vi "rm.server.open visualizer.vi"(8 "error in (no error)":errorcluster, 11 "Device Ref in":T1 format="%.0x") -> (0 "error out":errorcluster, 3 "reference out":refnum<vi>)   [LabVIEW 2016, in "RM.Server.lvlib"]
uses:
  RM.Server.lvlib
  <vilib>/NI Veristand/Custom Device API/Custom Device Item Ref.ctl
  rm.server.visualize.vi
  <vilib>/NI VeriStand/Custom Device API/Custom Device API.lvlib
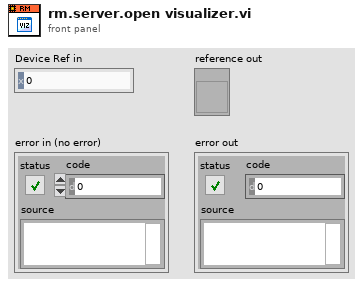
[diagram p1: front panel]
types:
  T1 = typedef "Custom Device API.lvlib/Custom Device Item Ref.ctl" = u64
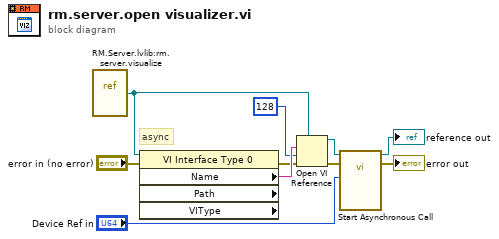
[diagram p0: block diagram]
diagram:
  # "async"
  n1 = vi-ref "RM.Server.lvlib:rm.server.visualize.vi"() -> (w10:refnum<vi>)
  n2 = property class="VI Interface Type 0" props=["Name", "Path", "VIType"](reference=w10, error in="error in (no error)") -> (error out=w5:errorcluster, "Name"=w9:string)  [unwired: 3 out]
  n3 = Open VI Reference(type specifier VI Refnum (for type only)=w10, vi path=w9, options=128, error in (no error)=w5) -> (vi reference=w1:refnum<vi>, error out=w4:errorcluster)  [unwired: 2 in]
  n4 = call-by-ref "Start Asynchronous Call"(reference=w1, error in=w4, "Item Ref in"="Device Ref in") -> (reference out=→"reference out":refnum<vi>, error out=→"error out":errorcluster)  [unwired: 9 in, 2 out]
